vi "Read Pixels and Copy to Display Image New.vi"(0 "fpga interface in":refnum<k20>, 5 "display channel number":i32, 7 "serial channel display parameters":T6[](array[typedef]) {"RAW parameters"."bayer parameters"."blue gain" format="%_4g"; "RAW parameters"."bayer parameters"."green gain" format="%_4g"; "RAW parameters"."bayer parameters"."red gain" format="%_4g"; "RAW parameters"."bayer parameters"."algorithm" items=["Bilinear", "VNG"]; "RAW parameters"."bayer parameters"."pattern" items=["GB", "GR", "BG", "RG"]}, 9 "image metadata":T4, 11 "error in (no error)":errorcluster) -> (4 "fpga interface out":refnum<k20>, 6 "display image":T3, 8 "output cluster":T2, 15 "error out":errorcluster)   [LabVIEW 2026]
uses:
  Types/Serial Channel Display Parameters.ctl
  <vilib>/vision/Image Controls.llb/IMAQ Image.ctl
  Types/RAW Interpretation for Display.ctl
  automotive-interface-plugins/src/labview/auto-vision/Automotive Vision/deps/NI148X/Getting Started/FPGA/Common/Types/Image Metadata.ctl
  <instrlib>/FlexRIO/CSI-2/v2/Common/Types/LLP Data Type.ctl
  GettingStarted_Common_148X_Host.lvlib
  <instrlib>/FlexRIO/CSI-2/v2/Common/NI CSI-2 API Common v2.lvlib
  FPGA/Common/GettingStarted_Common_148X_FPGA.lvlib
panel:
  out "size(s)":i32
  in  "Image Metadata and Data":T2 {"RAW parameters"."bayer parameters"."blue gain" format="%_4g"; "RAW parameters"."bayer parameters"."green gain" format="%_4g"; "RAW parameters"."bayer parameters"."red gain" format="%_4g"; "RAW parameters"."bayer parameters"."algorithm" items=["Bilinear", "VNG"]; "RAW parameters"."bayer parameters"."pattern" items=["GB", "GR", "BG", "RG"]}
  out "Array":u8[](array[numeric])
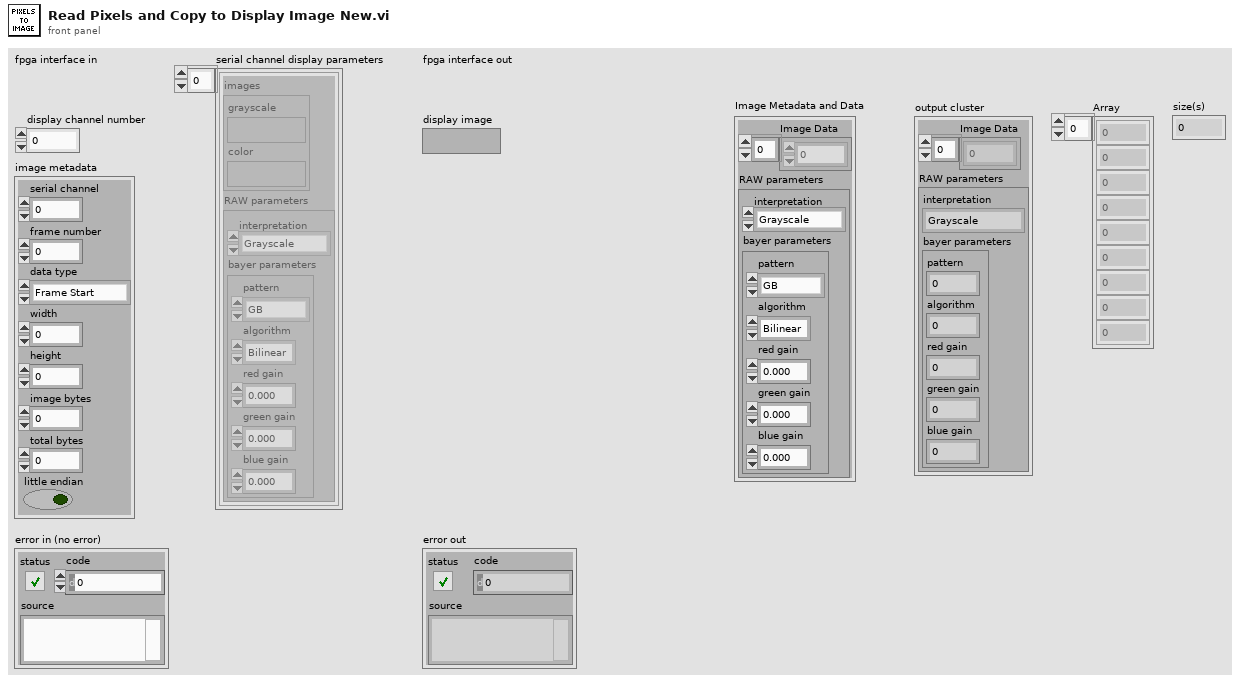
[diagram p1: front panel]
types:
  T1 = typedef "GettingStarted_Common_148X_Host.lvlib/RAW Interpretation for Display.ctl" = enum16{"Grayscale", "Bayer", "RGB", "YUV422", "YUV420", "Legacy YUV420"}
  T2 = cluster{"Image Data":u8[], "RAW parameters":cluster{"interpretation":T1, "bayer parameters":cluster{"pattern":i32, "algorithm":i32, "red gain":dbl, "green gain":dbl, "blue gain":dbl}}}
  T3 = typedef "IMAQ Image.ctl" = refnum<image>
  T4 = typedef "GettingStarted_Common_148X_FPGA.lvlib/Image Metadata.ctl" = cluster{"serial channel":fxp<+,3,3>, "frame number":u16, "data type":T5, "width":u16, "height":u16, "image bytes":u32, "total bytes":u32, "little endian":bool}
  T5 = typedef "NI CSI-2 API Common v2.lvlib/LLP Data Type.ctl" = enum8{"Frame Start", "Frame End", "Line Start", "Line End", "End of Transmission", "Reserved 0", "Reserved 1", "Reserved 2", "Generic Short Packet 1", "Generic Short Packet 2", "Generic Short Packet 3", "Generic Short Packet 4", "Generic Short Packet 5", "Generic Short Packet 6", "Generic Short Packet 7", "Generic Short Packet 8", "Null", "Blanking Data", "Embedded 8-bit non Image Data", "Generic Long Packet 1", "Generic Long Packet 2", "Generic Long Packet 3", "Generic Long Packet 4", "Reserved 3", "YUV420 8-bit", "YUV420 10-bit", "Legacy YUV420 8-bit", "Reserved 4", "YUV420 8-bit Chroma Shifted", "YUV420 10-bit Chroma Shifted", "YUV422 8-bit", "YUV422 10-bit", "RGB444", "RGB555", "RGB565", "RGB666", "RGB888", "Reserved 5", "Reserved 6", "RAW 24", "RAW 6", "RAW 7", "RAW 8", "RAW 10", "RAW 12", "RAW 14", "RAW 16", "RAW 20", "User Defined 8-bit Data 1", "User Defined 8-bit Data 2", "User Defined 8-bit Data 3", "User Defined 8-bit Data 4", "User Defined 8-bit Data 5", "User Defined 8-bit Data 6", "User Defined 8-bit Data 7", "User Defined 8-bit Data 8", "USL Command", "Reserved 7", "Reserved 8", "Reserved 9", "Reserved 10", "Reserved 11", "Reserved 12", "LRTE EPD Spacer"}
  T6 = typedef "GettingStarted_Common_148X_Host.lvlib/Serial Channel Display Parameters.ctl" = cluster{"images":cluster{"grayscale":T3, "color":T3}, "RAW parameters":cluster{"interpretation":T1, "bayer parameters":cluster{"pattern":i32, "algorithm":i32, "red gain":dbl, "green gain":dbl, "blue gain":dbl}}}
  T7 = cluster{"interpretation":T1, "bayer parameters":cluster{"pattern":i32, "algorithm":i32, "red gain":dbl, "green gain":dbl, "blue gain":dbl}}
  T8 = cluster{"pattern":i32, "algorithm":i32, "red gain":dbl, "green gain":dbl, "blue gain":dbl}
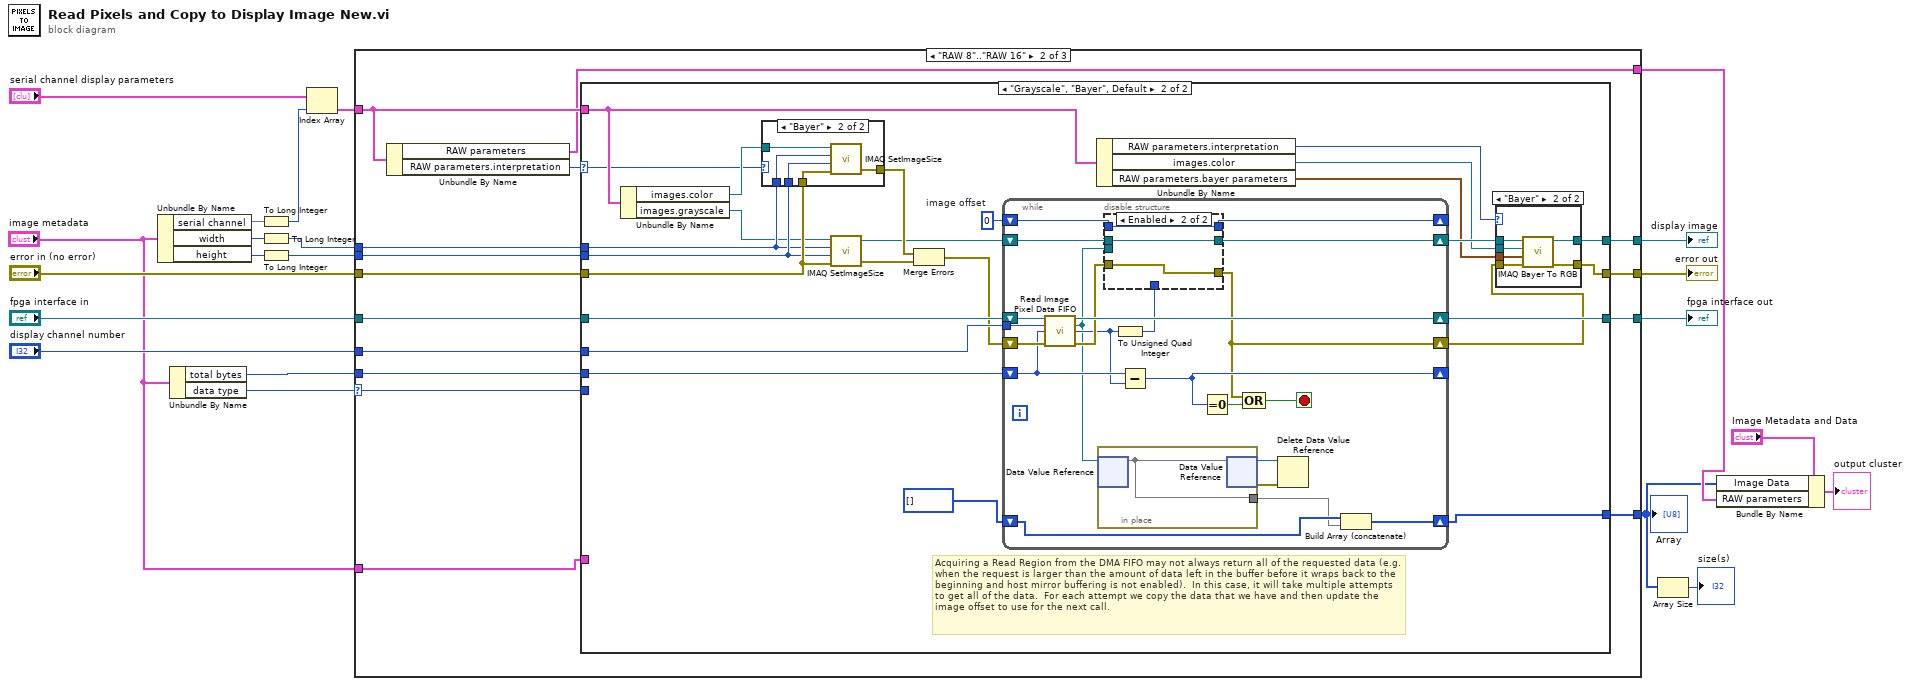
[diagram p0: block diagram]
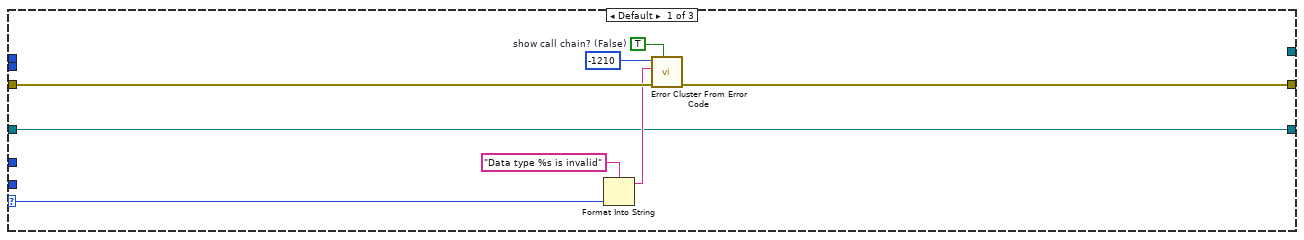
[diagram p2: hidden frame]
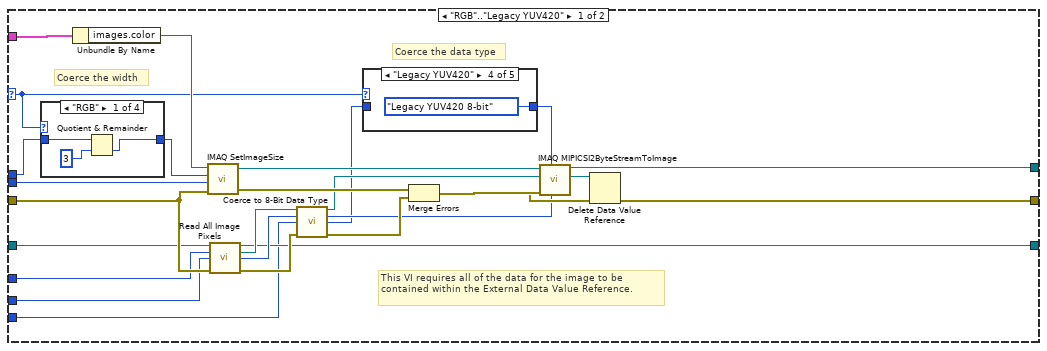
[diagram p3: hidden frame]
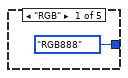
[diagram p4: hidden frame]
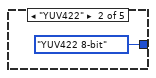
[diagram p5: hidden frame]
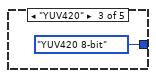
[diagram p6: hidden frame]
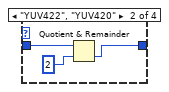
[diagram p8: hidden frame]
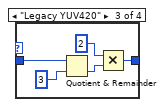
[diagram p9: hidden frame]
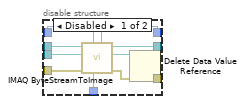
[diagram p12: hidden frame]
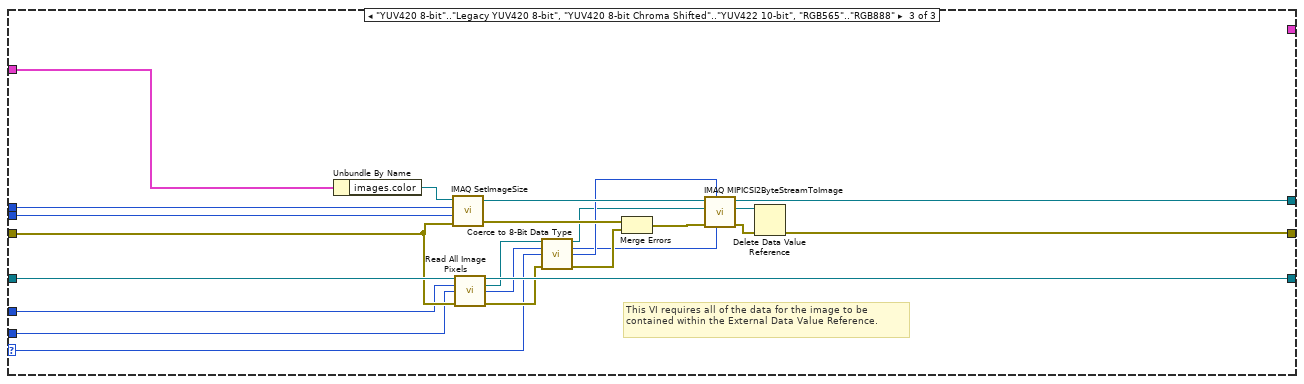
[diagram p14: hidden frame]
diagram:
  n1 = Unbundle By Name("image metadata") -> ("serial channel"=w18:fxp<+,3,3>, "width"=w15:u16, "height"=w16:u16)
  n2 = Unbundle By Name("image metadata") -> ("total bytes"=w21:u32, "data type"=w7:T5)
  n3 = To Long Integer(number=w18) -> (32bit integer=w17:i32)
  n4 = To Long Integer(number=w15) -> (32bit integer=w12:i32)
  n5 = To Long Integer(number=w16) -> (32bit integer=w13:i32)
  n6 = Index Array(array="serial channel display parameters", index=w17) -> (element=w9:T6)
  n7 = case shown="\"RAW 8\"..\"RAW 16\"" w7 {
    selector: w7 -> [w24 w34 w168]
    tunnel: w21 -> [_ w45 w178]
    tunnel: [w23 w44 w180] -> w20
    tunnel: "display channel number" -> [_ w43 w177]
    tunnel: "error in (no error)" -> [w28 w42 w181]
    tunnel: w13 -> [_ w41 w188]
    tunnel: w12 -> [_ w40 w187]
    tunnel: [_ w39 w176] -> w11
    tunnel: [w27 w38 w173] -> w10
    tunnel: w9 -> [_ w36 w185]
    tunnel: "fpga interface in" -> [w23 w37 w184]
    tunnel: [_ w33 _] -> w2
    tunnel: "image metadata" -> [_ w32 _]
    tunnel: [_ w31 _] -> w4
    frame Default {
      w29 = TRUE  # show call chain? (False)
      n8 = Format Into String(format string="Data type %s is invalid" ("error message (\"\")"), w24) -> (resulting string=w25:string)  [unwired: 2 in, 1 out]
      n9 = call <vilib>:"Error Cluster From Error Code.vi"("show call chain? (False)"=w29, "error in (no error)"=w28, "error message (\"\")"=w25, "error code (0)"=-1210) -> ("error out"=w27:errorcluster)  [unwired: 5 in]
    }
    frame "RAW 8".."RAW 16" {
      n10 = Unbundle By Name(w36) -> ("RAW parameters"=w31:T7, "RAW parameters.interpretation"=w35:T1)
      n11 = case shown="\"Grayscale\", \"Bayer\", Default" w35 {
        selector: w35 -> [w48 w92]
        tunnel: w45 -> [w55 w114]
        tunnel: [w59 w112] -> w44
        tunnel: w43 -> [w54 w111]
        tunnel: w42 -> [w60 w110]
        tunnel: w41 -> [w51 w108]
        tunnel: w40 -> [w50 w107]
        tunnel: [w57 w104] -> w39
        tunnel: [w58 w102] -> w38
        tunnel: w36 -> [w53 w97]
        tunnel: w37 -> [w56 w96]
        tunnel: w34 -> [w52 _]
        tunnel: [_ w90] -> w33
        tunnel: w32 -> [_ _]
        frame "RGB".."Legacy YUV420" {
          # "Coerce the data type"
          # "Coerce the width"
          # "This VI requires all of the data for the image to be contained within the External Data Value Reference."
          n12 = case shown="\"RGB\"" w48 {
            tunnel: w50 -> [w79 w82 w88 w89]
            tunnel: [w78 w81 w85 w89] -> w49
            frame "RGB" {
              n13 = Quotient & Remainder(x=w79, y=3) -> (floor(x/y)=w78:i32)  [unwired: 1 out]
            }
            frame "YUV422", "YUV420" {
              n14 = Quotient & Remainder(x=w82, y=2) -> (floor(x/y)=w81:i32)  [unwired: 1 out]
            }
            frame "Legacy YUV420" {
              n15 = Quotient & Remainder(x=w88, y=3) -> (floor(x/y)=w86:i32)  [unwired: 1 out]
              n16 = Multiply(x=2, y=w86) -> (x*y=w85:i32)
            }
            frame Default {
            }
          }
          n17 = Unbundle By Name(w53) -> ("images.color"=w72:T3)
          n18 = call "IMAQ SetImageSize"("error in (no error)"=w60, "Y Resolution"=w51, "X Resolution"=w49, "Image"=w72) -> ("error out"=w70:errorcluster, "Image Out"=w71:T3)  [unwired: 1 in]
          n19 = call "Read All Image Pixels.vi"("fpga inteface in"=w56, "display channel number"=w54, "image bytes"=w55, "error in (no error)"=w60) -> ("fpga interface out"=w59:refnum<k20>, "image pixel data region"=w65:refnum<data-value>, "elements in region"=w64:u32, "error out"=w66:errorcluster)  [unwired: 8 in]
          n20 = call "Coerce to 8-Bit Data Type.vi"("image pixel data region in"=w65, "image bytes in"=w64, "data type in"=w52, "error in (no error)"=w66) -> ("image pixel data region out"=w61:refnum<data-value>, "image bytes out"=w62:u32, "data type out"=w46:T5, "error out"=w63:errorcluster)  [unwired: 8 in]
          n21 = case shown="\"Legacy YUV420\"" w48 {
            tunnel: w46 -> [_ _ _ _ w77]
            tunnel: [LLP_Data_Type."RGB888" ("data type") LLP_Data_Type."YUV422 8-bit" ("data type") LLP_Data_Type."YUV420 8-bit" ("data type") LLP_Data_Type."Legacy YUV420 8-bit" ("data type") w77] -> w47
            frame "RGB" {
            }
            frame "YUV422" {
            }
            frame "YUV420" {
            }
            frame "Legacy YUV420" {
            }
            frame Default {
            }
          }
          n22 = Merge Errors(w70, w63) -> (w69:errorcluster)
          n23 = call "IMAQ MIPICSI2ByteStreamToImage"("Bytes to Copy"=w62, "Format"=w47, "error in (no error)"=w69, "Byte Stream In"=w61, "Image In"=w71) -> ("error out"=w68:errorcluster, "Byte Stream Out"=w67:refnum<data-value>, "Image Out"=w57:T3)  [unwired: 3 in, 1 out]
          n24 = Delete Data Value Reference(data value reference=w67, error in=w68) -> (error out=w58:errorcluster)  [unwired: 1 out]
        }
        frame "Grayscale", "Bayer", Default {
          w93 = u32 0  # image offset
          # "Acquiring a Read Region from the DMA FIFO may not always return all of the requested data (e.g. when the request is larger than the amount of data left in the buffer before it wraps back to the beginning and host mirror buffering is not enabled).  In this case, it will take multiple attempts to get all of the data.  For each attempt we copy the data that we have and then update the image offset to use for the next call."
          n25 = Unbundle By Name(w97) -> ("images.color"=w106:T3, "images.grayscale"=w101:T3)
          n26 = case shown="\"Bayer\"" w92 {
            tunnel: w110 -> [w115 w120]
            tunnel: [w115 w119] -> w109
            tunnel: w106 -> [_ w118]
            tunnel: w108 -> [_ w117]
            tunnel: w107 -> [_ w116]
            frame "Grayscale", Default {
            }
            frame "Bayer" {
              n27 = call "IMAQ SetImageSize"("error in (no error)"=w120, "Y Resolution"=w117, "X Resolution"=w116, "Image"=w118) -> ("error out"=w119:errorcluster)  [unwired: 1 in, 1 out]
            }
          }
          n28 = call "IMAQ SetImageSize"("error in (no error)"=w110, "Y Resolution"=w108, "X Resolution"=w107, "Image"=w101) -> ("error out"=w113:errorcluster, "Image Out"=w95:T3)  [unwired: 1 in]
          n29 = Merge Errors(w109, w113) -> (w94:errorcluster)
          n30 = while {
            tunnel: w111 -> [w140]
            shift-right: [w141] -> w112
            shift-left: w96 -> [w142]
            shift-right: [w129] -> w103
            shift-left: w94 -> [w139]
            shift-right: [w137] -> w105
            shift-left: w95 -> [w138]
            shift-right: [w132] -> _
            shift-left: w114 -> [w134]
            shift-right: [w128] -> _
            shift-left: w93 -> [w127]
            shift-right: [w121] -> w90
            shift-left: u8[] [] -> [w123]
            stop <- w130 stop-if-true
            n31 = call "Read Image Pixel Data FIFO.vi"("fpga inteface in"=w142, "display channel number"=w140, "number of elements"=w134, "error in (no error)"=w139) -> ("fpga interface out"=w141:refnum<k20>, "image pixel data region"=w126:refnum<data-value>, "elements in region"=w133:u32, "error out"=w136:errorcluster)  [unwired: 7 in, 1 out]
            n32 = in-place {
              in-place-border: [w156] -> w122
              n33 = in-place-dvr #1(w126) -> (w156:u8[])  [unwired: 1 out]
              n34 = in-place-dvr #1(w156) -> (w124:refnum<data-value>, w125:errorcluster)
            }
            n35 = To Unsigned Quad Integer(1:w133) -> (0:w135:u64)
            n36 = disable-structure shown="Enabled" {
              disable-tunnel: w138 -> [w152 w155]
              disable-tunnel: [w151 w155] -> w137
              disable-tunnel: w136 -> [w150 w154]
              disable-tunnel: w135 -> [w149 _]
              disable-tunnel: [w146 w154] -> w129
              disable-tunnel: [w145 w153] -> w128
              disable-tunnel: w127 -> [w144 w153]
              disable-tunnel: w126 -> [w143 _]
              frame Disabled {
                n37 = call "IMAQ ByteStreamToImage"("Bytes to Copy"=w149, "Image Byte Offset In"=w144, "error in (no error)"=w150, "Byte Stream In"=w143, "Image In"=w152) -> ("error out"=w147:errorcluster, "Byte Stream Out"=w148:refnum<data-value>, "Image Out"=w151:T3, "Image Byte Offset Out"=w145:u32)  [unwired: 2 in, 1 out]
                n38 = Delete Data Value Reference(data value reference=w148, error in=w147) -> (error out=w146:errorcluster)  [unwired: 1 out]
              }
              frame Enabled {
              }
            }
            n39 = Subtract(x=w134, y=w133) -> (x-y=w132:u32)
            n40 = Equal To 0?(x=w132) -> (x = 0?=w131:bool)
            n41 = Compound Arithmetic op=OR(w129, w131) -> (w130:bool)
            n42 = Delete Data Value Reference(data value reference=w124, error in=w125) -> ()  [unwired: 2 out]
            n43 = Build Array (concatenate)(w123, w122) -> (w121:u8[])
          }
          n44 = Unbundle By Name(w97) -> ("RAW parameters.interpretation"=w98:T1, "images.color"=w99:T3, "RAW parameters.bayer parameters"=w100:T8)
          n45 = case shown="\"Bayer\"" w98 {
            tunnel: w105 -> [w157 w164]
            tunnel: [w157 w163] -> w104
            tunnel: w103 -> [w158 w162]
            tunnel: [w158 w161] -> w102
            tunnel: w99 -> [_ w160]
            tunnel: w100 -> [_ w159]
            frame "Grayscale", Default {
            }
            frame "Bayer" {
              n46 = call "IMAQ Bayer To RGB"("error in (no error)"=w162, "Bayer Parameters"=w159, "Image Dst"=w160, "Image Src"=w164) -> ("error out"=w161:errorcluster, "Image Dst Out"=w163:T3)  [unwired: 6 in]
            }
          }
        }
      }
    }
    frame "YUV420 8-bit".."Legacy YUV420 8-bit", "YUV420 8-bit Chroma Shifted".."YUV422 10-bit", "RGB565".."RGB888" {
      # "This VI requires all of the data for the image to be contained within the External Data Value Reference."
      n47 = Unbundle By Name(w185) -> ("images.color"=w186:T3)
      n48 = call "IMAQ SetImageSize"("error in (no error)"=w181, "Y Resolution"=w188, "X Resolution"=w187, "Image"=w186) -> ("error out"=w182:errorcluster, "Image Out"=w183:T3)  [unwired: 1 in]
      n49 = call "Read All Image Pixels.vi"("fpga inteface in"=w184, "display channel number"=w177, "image bytes"=w178, "error in (no error)"=w181) -> ("fpga interface out"=w180:refnum<k20>, "image pixel data region"=w171:refnum<data-value>, "elements in region"=w170:u32, "error out"=w172:errorcluster)  [unwired: 8 in]
      n50 = call "Coerce to 8-Bit Data Type.vi"("image pixel data region in"=w171, "image bytes in"=w170, "data type in"=w168, "error in (no error)"=w172) -> ("image pixel data region out"=w165:refnum<data-value>, "image bytes out"=w166:u32, "data type out"=w167:T5, "error out"=w169:errorcluster)  [unwired: 8 in]
      n51 = Merge Errors(w182, w169) -> (w179:errorcluster)
      n52 = call "IMAQ MIPICSI2ByteStreamToImage"("Bytes to Copy"=w166, "Format"=w167, "error in (no error)"=w179, "Byte Stream In"=w165, "Image In"=w183) -> ("error out"=w175:errorcluster, "Byte Stream Out"=w174:refnum<data-value>, "Image Out"=w176:T3)  [unwired: 3 in, 1 out]
      n53 = Delete Data Value Reference(data value reference=w174, error in=w175) -> (error out=w173:errorcluster)  [unwired: 1 out]
    }
  }
  "display image" <- w11
  "fpga interface out" <- w20
  "error out" <- w10
  "Array" <- w2
  n54 = Array Size(array=w2) -> (size(s)=→"size(s)":i32)
  n55 = Bundle By Name(cluster="Image Metadata and Data", "Image Data"=w2, "RAW parameters"=w4) -> (→"output cluster":T2)
